vi "Find Average Center.vi"(5 "Position":i32, 7 "Tray Number":i32, 9 "XYZTheta":dbl[](array[numeric]), 11 "Gantry In":refnum<k24>) -> (1 "XYZTheta":dbl[](array[numeric]) format="%.6g", 3 "Gantry Out":refnum<k24>)   [LabVIEW 2020, in "Component Tray.lvclass"]
uses:
  Component Tray.lvclass
  Controller/Camera/Edmund Optics/Edmund Optics.lvclass
  Controller/Camera/Camera.lvclass
  Controller/Motion/A3200/A3200.lvclass
  Controller/Motion/Motion.lvclass
  Find Component.ctl
  Controller/Camera/Machine Vision.ctl
  C:/Program Files (x86)/Aerotech/A3200/LabVIEW/2010/Bin/Aerotech.A3200.dll
  Program Files (x86)/Aerotech/A3200/LabVIEW/2010/Bin/Aerotech.A3200.dll
  Controller/Camera/Camera settings.ctl
  Controller/Camera/Image processing.ctl
  Controller/Camera/Material.ctl
panel:
  out "Program Stopped":bool
  out "XY Graph":cluster{"X":dbl, "Y":dbl}[](graph)
  out "Sensor ID Location":dbl[](array[numeric])
  in  "Go to Sensor ID":bool
  out "CH1 Location":dbl[](array[numeric])
  in  "Verify CH1":bool
  out "CH1 correct?":bool
  in  "Go to CH1":bool
  in  "Focus step size":dbl format="%#_13g"
  in  "number of focus steps":i32
  out "Average Strength":dbl
  in  "Focus":bool
  in  "Material":T1
  out "All fiducials recorded":bool
  in  "Override presets":bool
  in  "Camera settings":T2={"Gamma"=1.6, "Gain"=0, "Sharpness"=0, "Contrast"=0.0, "Exposure"=0.0078125} {"Exposure" min=0.000244140625 max=0.5 scale=0.0002..0.5; "Contrast" min=0.0 max=1.0 scale=0.001..1.0; "Sharpness" min=0 max=2 step=1 scale=0.0..2.0; "Gain" min=0 max=100 step=1 scale=0.1..100.0; "Gamma" min=0.01 max=10.0 scale=0.01..10.0}
  in  "Image processing":T3={"Brightness"=128.0, "Contrast"=45.0, "Gamma"=1.0471123} {"Brightness" scale=0.0..400.0; "Contrast" scale=0.0..90.0; "Gamma" scale=0.005..5.0}
  in  "Machine Vision":T4
  out "Gantry":dbl[](array[numeric]) format="%.6g"
  out "Sum":dbl[](array[numeric]) format="%.6g"
  out "CH197 XY":dbl[](array[numeric]) format="%.6g"
  out "CH7 XY":dbl[](array[numeric]) format="%.6g"
  out "CH191 XY":dbl[](array[numeric]) format="%.6g"
  out "CH2 XY":dbl[](array[numeric]) format="%.6g"
  in  "Record CH7":bool
  in  "Record CH197":bool
  in  "Record CH191":bool
  in  "Record CH2":bool
  in  "Go to CH197":bool
  in  "Go to CH7":bool
  in  "Go to CH191":bool
  in  "Go to CH2":bool
  in  "Joystick":bool
  out "Camera":dbl[](array[numeric]) format="%.6g"
  in  "Go to Center":bool
  in  "Component":T5
  in  "Stop Program":bool
  out "Image":T6(plugin-control)
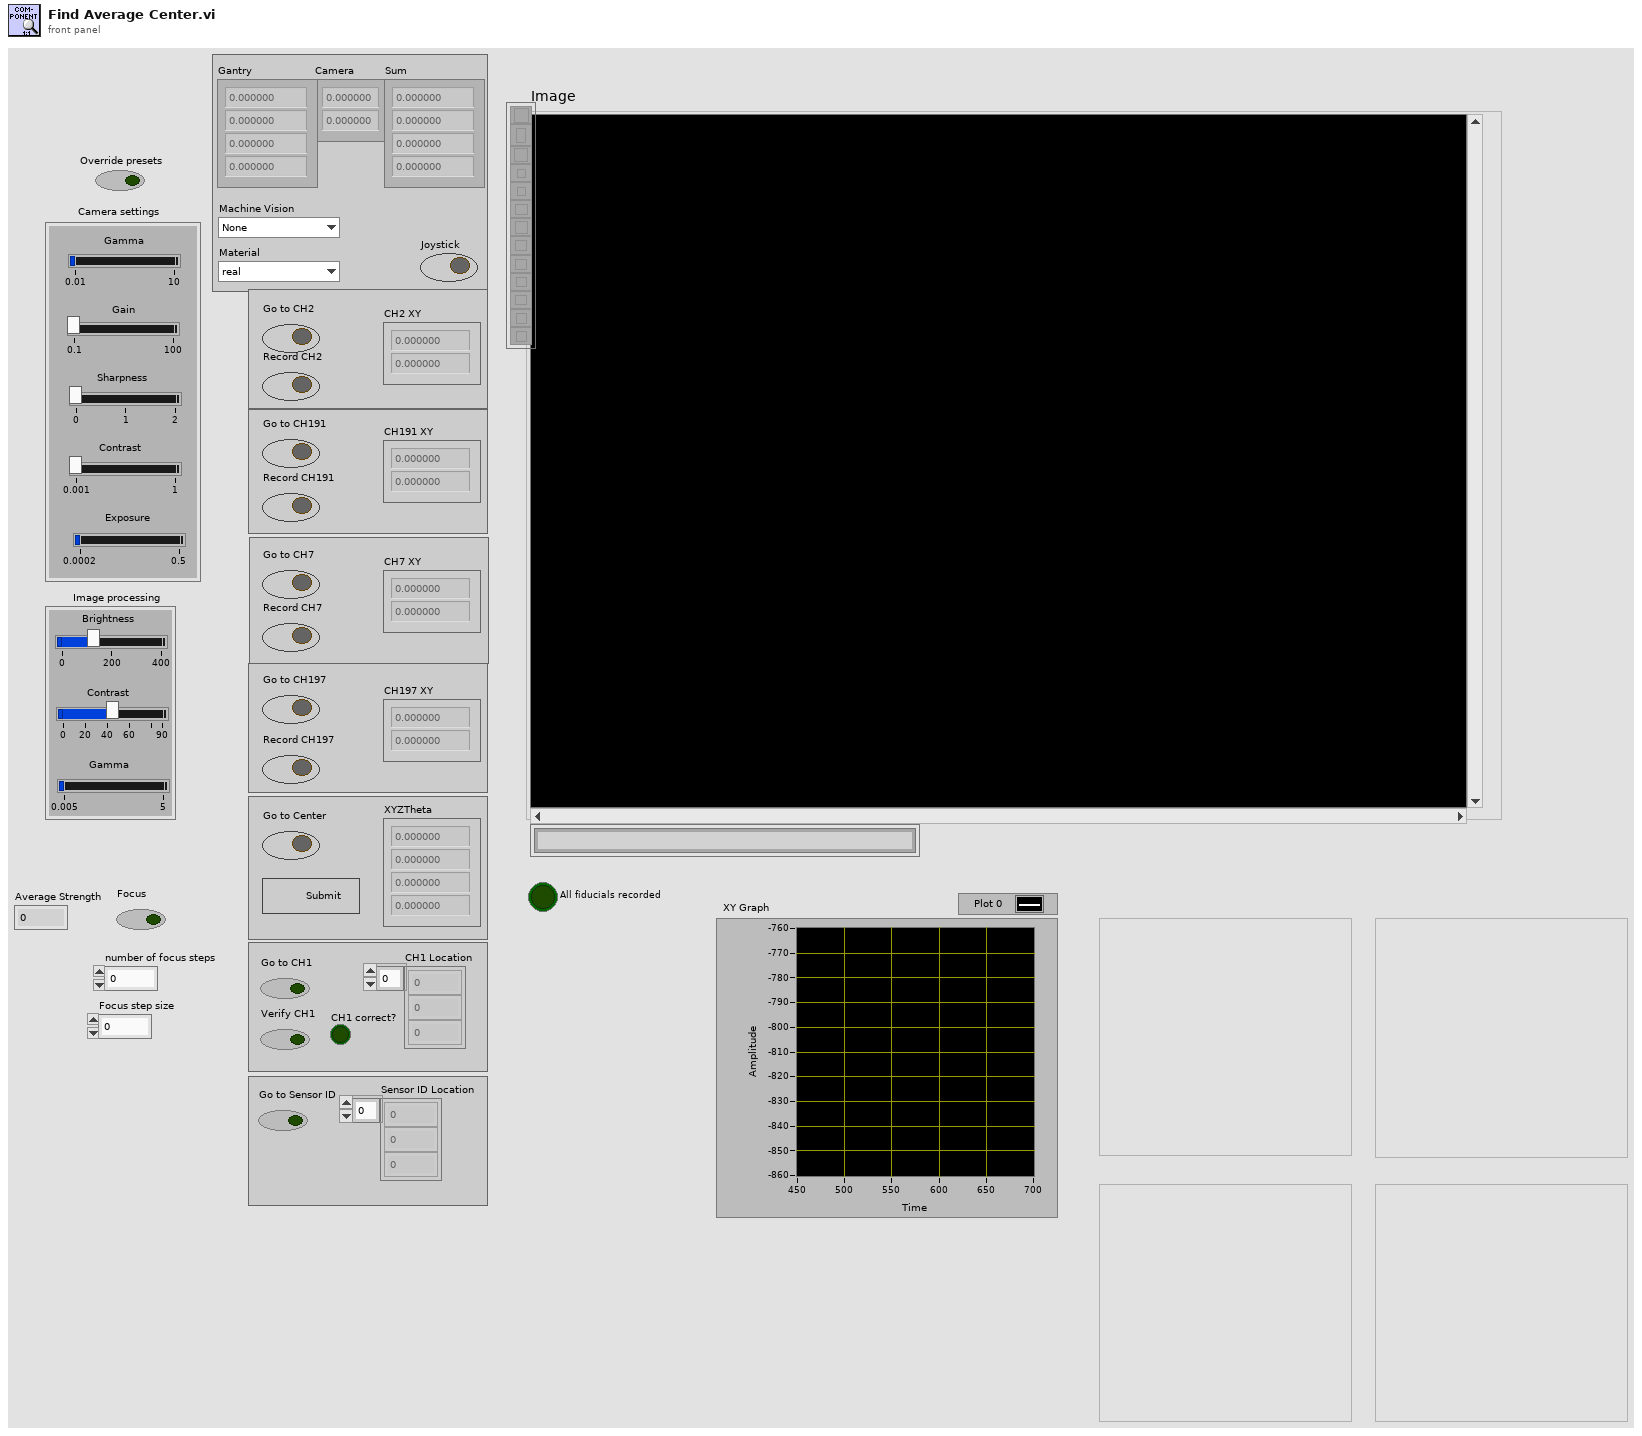
[diagram p1: front panel]
types:
  T1 = typedef "Camera.lvclass/Material.ctl" = enum16{"real", "dummy", "PETG"}
  T2 = typedef "Camera.lvclass/Camera settings.ctl" = cluster{"Gamma":dbl, "Gain":i64, "Sharpness":i64, "Contrast":dbl, "Exposure":dbl}
  T3 = typedef "Camera.lvclass/Image processing.ctl" = cluster{"Brightness":sgl, "Contrast":sgl, "Gamma":sgl}
  T4 = typedef "Camera.lvclass/Machine Vision.ctl" = enum16{"None", "Tray Fiducials", "HPK Silicon", "100um dot", "Hexaboard", "Corner (TL, BR)", "Corner (BL, TR)", "BP gold pad 1", "BP gold pad 2", "BP gold pad 3", "dummy sensor CH2", "dummy sensor CH7", "dummy sensor CH191", "dummy sensor CH197", "sensor box", "sensor circle", "PCB PETG CH2", "PCB PETG CH7", "PCB PETG CH191", "PCB PETG CH197"}
  T5 = typedef "Component Tray.lvclass/Find Component.ctl" = cluster{"New Fiducials":dbl[], "Past Fiducials":dbl[], "XYZTheta":dbl[], "Fiducials Path":path, "Position":i32, "CH1 Location":dbl[], "Sensor ID Location":dbl[]}
  T6 = typedef "IMAQ Image.ctl" = refnum<image>
  T7 = typedef "File Paths.ctl" = cluster{"Glue Pattern Folder":path, "Carrier Tray Folder":path, "Pick Up Tool Fixture Folder":path, "Components Folder":path, "Bellows Tool Offset.txt":path, "Pick Up Tool Offset.txt":path, "Dispense Tip Offset.txt":path, "Log Files":path, "Gantry Assembly Map.txt":path, "Syringe and offset map.txt":path}
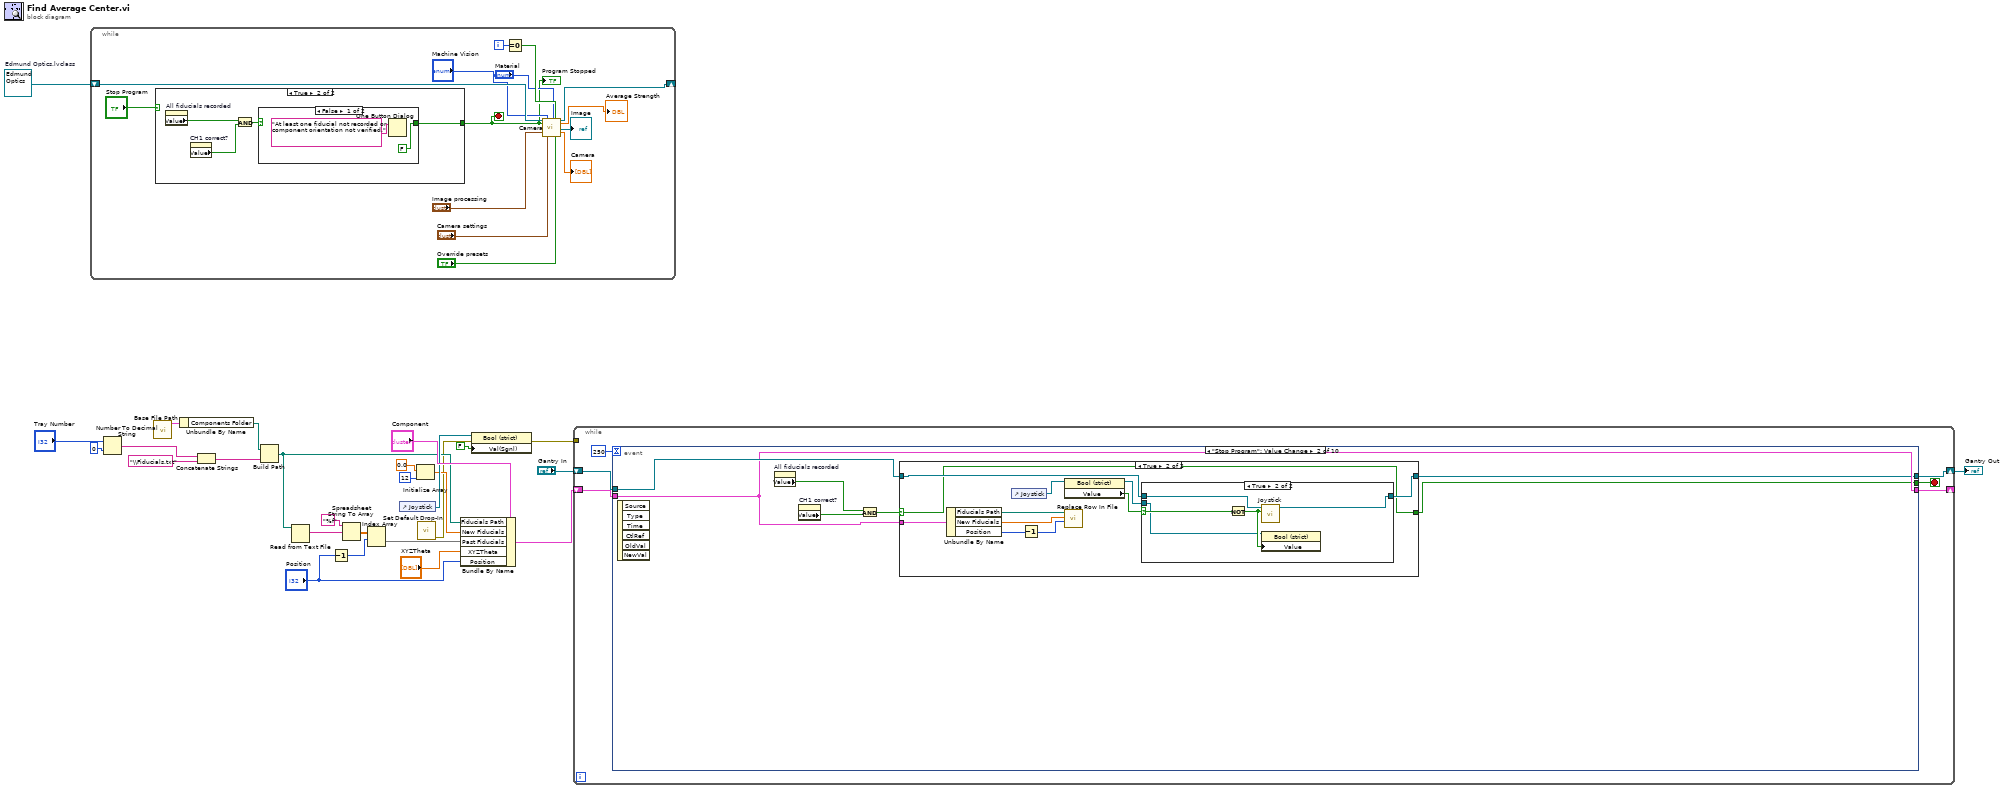
[diagram p0: block diagram]
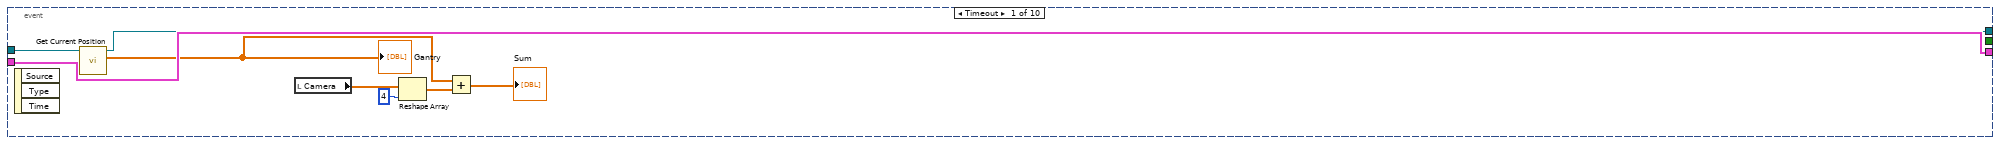
[diagram p2: hidden frame]
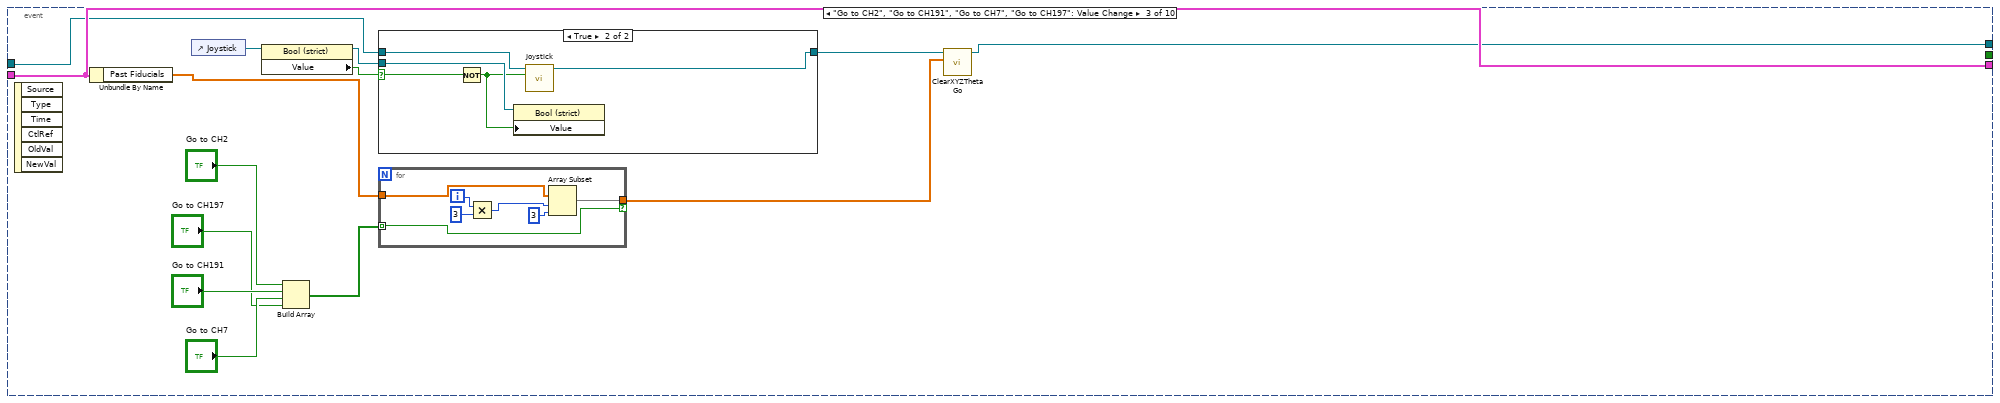
[diagram p5: hidden frame]
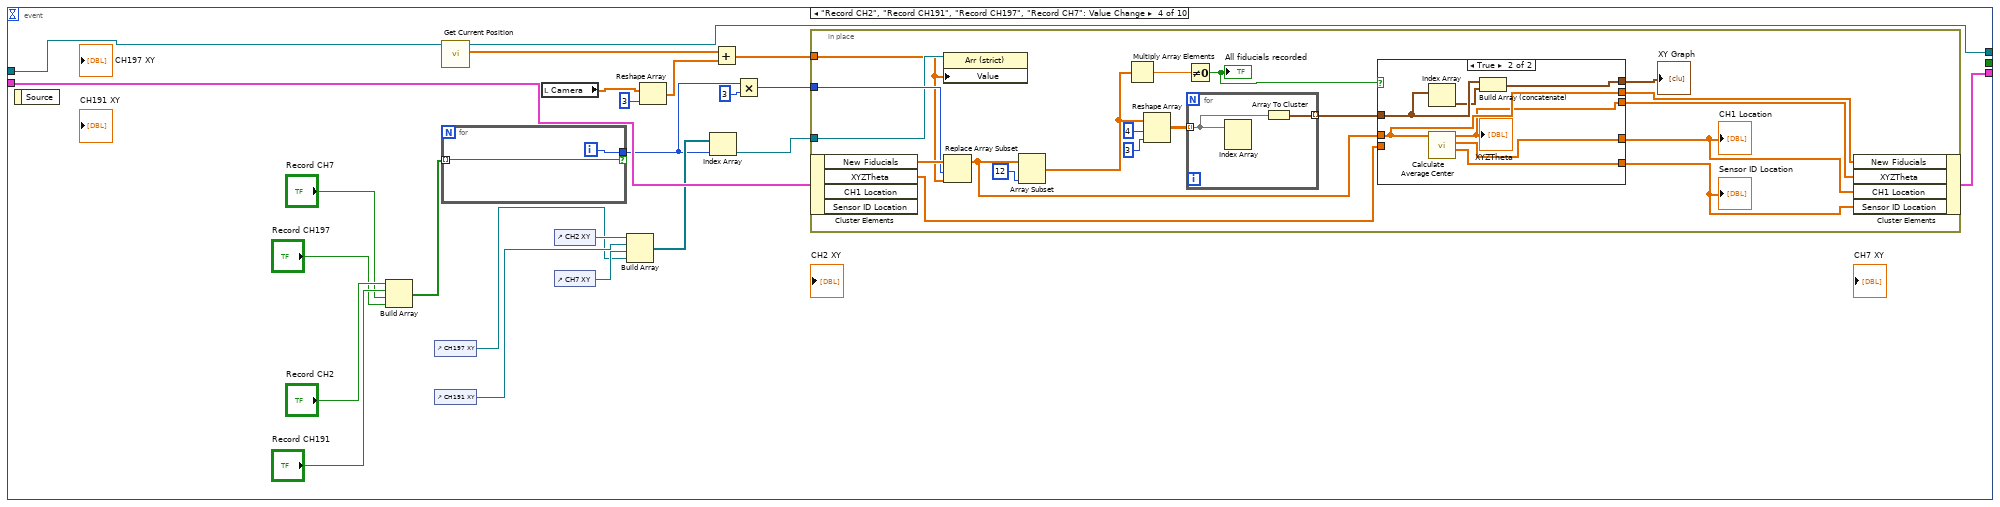
[diagram p7: hidden frame]
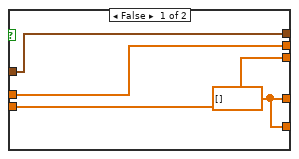
[diagram p8: hidden frame]
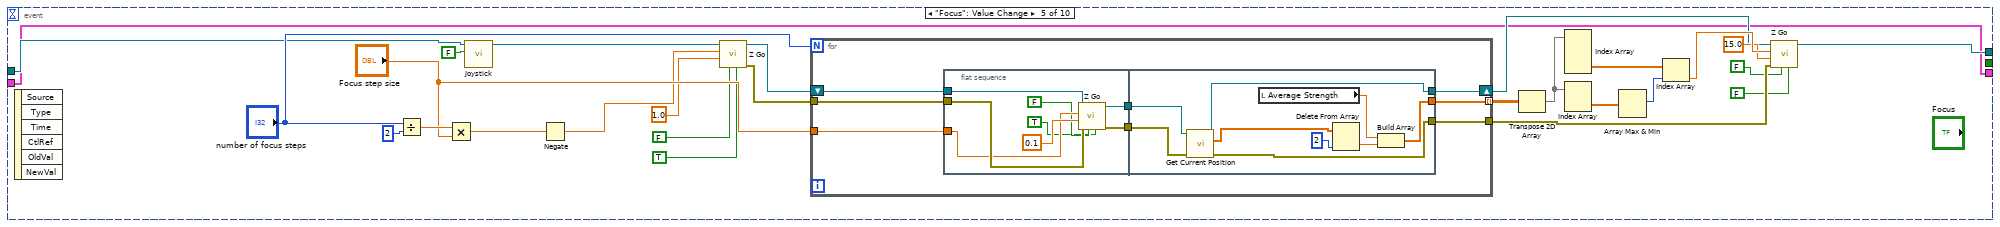
[diagram p9: hidden frame]
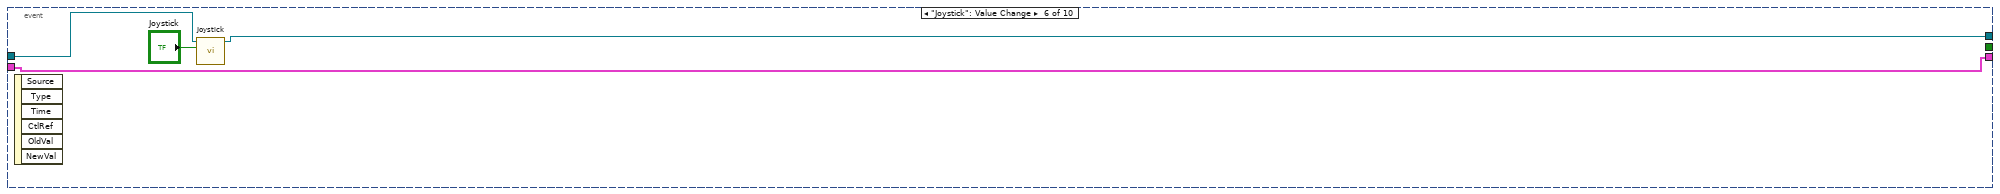
[diagram p10: hidden frame]
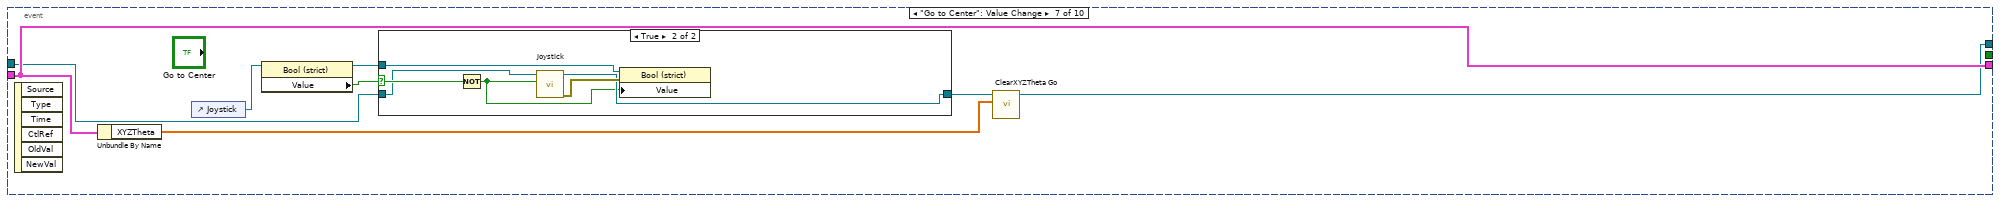
[diagram p11: hidden frame]
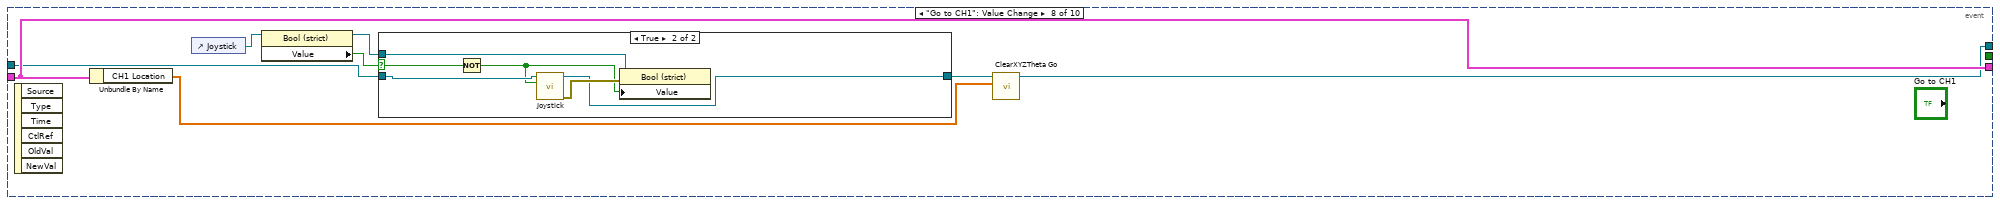
[diagram p13: hidden frame]
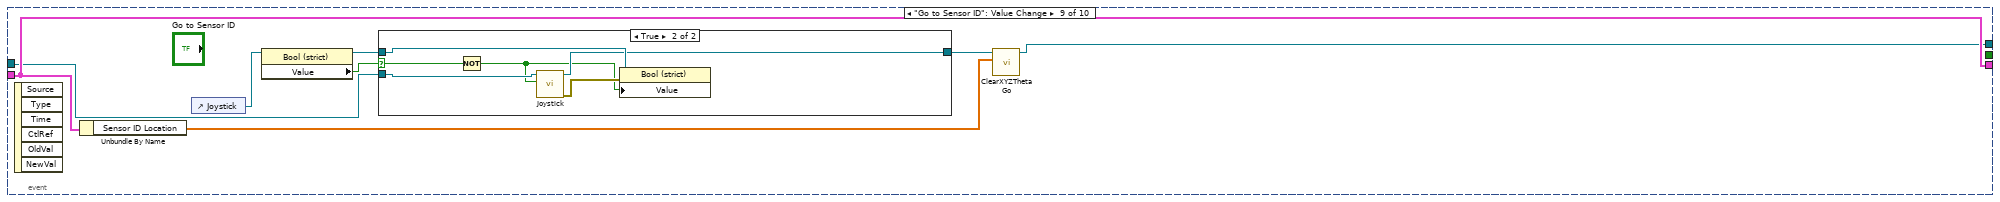
[diagram p15: hidden frame]
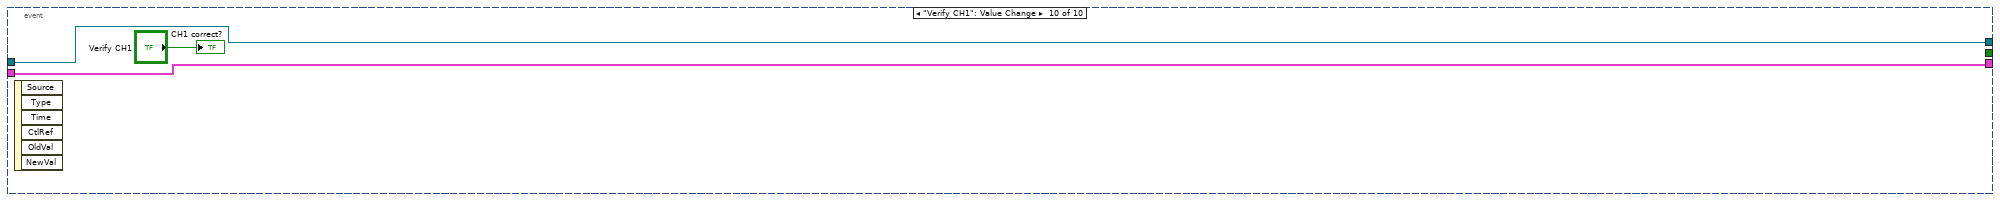
[diagram p17: hidden frame]
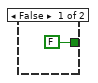
[diagram p18: hidden frame]
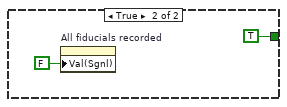
[diagram p19: hidden frame]
diagram:
  w22 = refnum<class "Edmund Optics.lvclass"> refnum  # Edmund Optics.lvclass
  n1 = while {
    shift-right: [w37] -> _
    shift-left: w22 -> [w41]
    i -> [w33]
    stop <- w28 stop-if-true
    n2 = case shown="True" "Stop Program" {
      tunnel: [FALSE w43] -> w28
      frame False {
      }
      frame True {
        n3 = property on="All fiducials recorded" class="Bool (strict)"() -> ("Value"=w46:bool)  [unwired: 2 in, 2 out]
        n4 = property on="CH1 correct?" class="Bool (strict)"() -> ("Value"=w44:bool)  [unwired: 2 in, 2 out]
        n5 = And(x=w46, y=w44) -> (x .and. y?=w45:bool)
        n6 = case shown="False" w45 {
          tunnel: [FALSE TRUE] -> w43
          frame False {
            n7 = One Button Dialog(message="At least one fiducial not recorded or component orientation not verified.") -> ()  [unwired: 1 in, 1 out]
          }
          frame True {
            n8 = property on="All fiducials recorded" class="Bool (strict)"("Val(Sgnl)"=FALSE) -> ()  [unwired: 2 in, 2 out]
          }
        }
      }
    }
    "Program Stopped" <- w28
    n9 = Equal To 0?(x=w33) -> (x = 0?=w32:bool)
    n10 = call "Camera.vi"("Camera in"=w41, "Stop"=w28, "BCG Image Processing"="Image processing", "Machine Vision"="Machine Vision", "Camera settings"="Camera settings", "Material"="Material", "Loop 0"=w32, "Override presets"="Override presets") -> ("Camera out"=w37:refnum<class "Edmund Optics.lvclass">, "Average Strength"=→"Average Strength":dbl, "Image"=→"Image":T6, "Camera"=→"Camera":dbl[])  [unwired: 6 in, 2 out]
  }
  n11 = Number To Decimal String(number="Tray Number", width (-)=i16 0) -> (decimal integer string=w16:string)
  n12 = call "Base File Path.vi"() -> ("Paths Out"=w13:T7)  [unwired: 11 in]
  n13 = Unbundle By Name(w13) -> ("Components Folder"=w15:path)
  n14 = Concatenate Strings(w16, "\\Fiducials.txt" ("string")) -> (w18:string)
  n15 = Build Path(base path=w15, name or relative path=w18) -> (appended path=w7:path)
  n16 = Read from Text File(file (use dialog)=w7) -> (text=w19:string)  [unwired: 3 in, 3 out]
  n17 = Decrement(x="Position") -> (x-1=w4:i32)
  n18 = Spreadsheet String To Array(format string="%f", spreadsheet string=w19) -> (array=w21:dbl[][])  [unwired: 2 in]
  n19 = Index Array(array=w21, index (row)=w4) -> (element=w11:dbl[])  [unwired: 1 in]
  n20 = control-ref of="Joystick"() -> (w25:refnum<vi>)
  n21 = Initialize Array(0.0 ("element"), 12 ("dimension size")) -> (w10:dbl[])
  n22 = call "Set Default Drop-In.vi"() -> ("error out"=w3:errorcluster)  [unwired: 11 in]
  n23 = Bundle By Name(cluster="Component", "Fiducials Path"=w7, "New Fiducials"=w10, "Past Fiducials"=w11, "XYZTheta"="XYZTheta", "Position"="Position") -> (w26:T5)
  n24 = property class="Bool (strict)"(reference=w25, error in=w3, "Val(Sgnl)"=FALSE) -> (error out=w23:errorcluster)  [unwired: 1 out]
  n25 = while {
    shift-right: [w54] -> _
    shift-left: w26 -> [w55]
    tunnel: w23 -> [_]
    shift-right: [w51] -> w1
    shift-left: "Gantry In" -> [w52]
    stop <- w56 stop-if-true
    n26 = event shown="[1] \"Stop Program\": Value Change" {
      selector: _ -> [_ _ _ _ _ _ _ _ _ _]
      dyn-events: _ -> [_ _ _ _ _ _ _ _ _ _]
      timeout: 250 -> [_ _ _ _ _ _ _ _ _ _]
      tunnel: [_ w68 _ _ _ _ _ _ _ _] -> w56
      tunnel: w55 -> [w63 w70 w97 w140 w184 w230 w237 w252 w267 w277]
      tunnel: [w63 w70 w97 w139 w184 w230 w237 w252 w267 w277] -> w54
      tunnel: w52 -> [w59 w71 w94 w120 w186 w229 w233 w248 w263 w278]
      tunnel: [w58 w69 w91 w118 w185 w227 w231 w246 w261 w278] -> w51
      event Timeout {
        n27 = event-data() -> ()  [unwired: 1 in, 3 out]
        n28 = call "Get Current Position.vi"("Gantry In"=w59) -> ("XYZTheta Out"=w57:dbl[], "Gantry Out"=w58:refnum<k24>)  [unwired: 8 in, 1 out]
        "Gantry" <- w57
        n29 = local read "Camera"() -> (w62:dbl[])
        n30 = Reshape Array(w62, 4 ("dimension size")) -> (w60:dbl[])
        n31 = Add(x=w57, y=w60) -> (x+y=→"Sum":dbl[])
      }
      event "Stop Program": Value Change {
        n32 = event-data() -> ()  [unwired: 1 in, 6 out]
        n33 = property on="All fiducials recorded" class="Bool (strict)"() -> ("Value"=w66:bool)  [unwired: 2 in, 2 out]
        n34 = property on="CH1 correct?" class="Bool (strict)"() -> ("Value"=w67:bool)  [unwired: 2 in, 2 out]
        n35 = And(x=w66, y=w67) -> (x .and. y?=w65:bool)
        n36 = case shown="True" w65 {
          selector: w65 -> [w72 w81]
          tunnel: w71 -> [w73 w83]
          tunnel: w70 -> [_ w84]
          tunnel: [w73 w82] -> w69
          tunnel: [w72 w81] -> w68
          frame False {
          }
          frame True {
            n37 = Unbundle By Name(w84) -> ("Fiducials Path"=w78:path, "New Fiducials"=w77:dbl[], "Position"=w79:i32)
            n38 = control-ref of="Joystick"() -> (w75:refnum<vi>)
            n39 = Decrement(x=w79) -> (x-1=w80:i32)
            n40 = property class="Bool (strict)"(reference=w75) -> (reference out=w74:refnum<vi>, "Value"=w76:bool)  [unwired: 1 in, 1 out]
            n41 = call "Replace Row In File.vi"("Index"=w80, "Insert Array"=w77, "Path"=w78) -> ()  [unwired: 8 in, 1 out]
            n42 = case shown="True" w76 {
              selector: w76 -> [_ w90]
              tunnel: w83 -> [w85 w89]
              tunnel: [w85 w88] -> w82
              tunnel: w74 -> [_ w86]
              frame False {
              }
              frame True {
                n43 = Not(x=w90) -> (.not. x?=w87:bool)
                n44 = call "Joystick.vi"("Joystick"=w87, "Gantry In"=w89) -> ("Gantry Out"=w88:refnum<k24>)  [unwired: 8 in, 1 out]
                n45 = property class="Bool (strict)"(reference=w86, "Value"=w87) -> ()  [unwired: 1 in, 2 out]
              }
            }
          }
        }
      }
      event "Go to CH2", "Go to CH191", "Go to CH7", "Go to CH197": Value Change {
        n46 = event-data() -> ()  [unwired: 1 in, 6 out]
        n47 = Unbundle By Name(w97) -> ("Past Fiducials"=w99:dbl[])
        n48 = control-ref of="Joystick"() -> (w92:refnum<vi>)
        n49 = property class="Bool (strict)"(reference=w92) -> (reference out=w95:refnum<vi>, "Value"=w96:bool)  [unwired: 1 in, 1 out]
        n50 = Build Array("Go to CH2", "Go to CH191", "Go to CH7", "Go to CH197") -> (w100:bool[])
        n51 = case shown="True" w96 {
          selector: w96 -> [_ w110]
          tunnel: w94 -> [w105 w108]
          tunnel: [w105 w106] -> w93
          tunnel: w95 -> [_ w109]
          frame False {
          }
          frame True {
            n52 = Not(x=w110) -> (.not. x?=w107:bool)
            n53 = property class="Bool (strict)"(reference=w109, "Value"=w107) -> ()  [unwired: 1 in, 2 out]
            n54 = call "Joystick.vi"("Joystick"=w107, "Gantry In"=w108) -> ("Gantry Out"=w106:refnum<k24>)  [unwired: 8 in, 1 out]
          }
        }
        n55 = for {
          tunnel: w100 -> [w117] mode=indexing
          tunnel: w99 -> [w116]
          tunnel: [w111] -> w98 if=w117
          i -> [w114]
          n56 = Multiply(x=w114, y=3) -> (x*y=w112:i32)
          n57 = Array Subset(array=w116, index=w112, length=3) -> (w111:dbl[])
        }
        n58 = call "ClearXYZTheta Go.vi"("XYZTheta In"=w98, "Gantry In"=w93) -> ("Gantry Out"=w91:refnum<k24>)  [unwired: 7 in, 2 out]
      }
      event "Record CH2", "Record CH191", "Record CH197", "Record CH7": Value Change {
        n59 = event-data() -> ()  [unwired: 1 in, 1 out]
        n60 = Build Array("Record CH2", "Record CH191", "Record CH7", "Record CH197") -> (w134:bool[])
        n61 = control-ref of="CH197 XY"() -> (w130:refnum<vi>)
        n62 = control-ref of="CH191 XY"() -> (w132:refnum<vi>)
        n63 = call "Get Current Position.vi"("Gantry In"=w120) -> ("XYZTheta Out"=w119:dbl[], "Gantry Out"=w118:refnum<k24>)  [unwired: 8 in, 1 out]
        n64 = for {
          tunnel: w134 -> [w141] mode=indexing
          tunnel: [w142] -> w126 if=w141
          i -> [w142]
        }
        n65 = local read "Camera"() -> (w123:dbl[])
        n66 = control-ref of="CH2 XY"() -> (w133:refnum<vi>)
        n67 = control-ref of="CH7 XY"() -> (w131:refnum<vi>)
        n68 = Build Array(w133, w132, w131, w130) -> (w129:refnum<vi>[])
        n69 = Reshape Array(w123, 3 ("dimension size")) -> (w122:dbl[])
        n70 = Index Array(array=w129, index=w126) -> (element=w128:refnum<vi>)
        n71 = Add(x=w119, y=w122) -> (x+y=w121:dbl[])
        n72 = Multiply(x=w126, y=3) -> (x*y=w124:i32)
        n73 = in-place {
          in-place-border: w124 -> [w159]
          in-place-border: w128 -> [w157]
          in-place-border: w121 -> [w155]
          n74 = in-place-cluster #1(w140) -> ("New Fiducials"=w160:dbl[], "XYZTheta"=w156:dbl[])  [unwired: 2 out]
          n75 = property class="Arr (strict)"(reference=w157, "Value"=w155) -> ()  [unwired: 1 in, 2 out]
          n76 = Replace Array Subset(array=w160, new element=w155, index=w159) -> (w154:dbl[])
          n77 = Array Subset(array=w154, length=12) -> (w149:dbl[])  [unwired: 1 in]
          n78 = Multiply Array Elements(1:w149) -> (0:w152:dbl)
          n79 = Reshape Array(w149, 4 ("dimension size"), 3 ("dimension size")) -> (w146:dbl[][])
          n80 = Not Equal To 0?(x=w152) -> (x != 0?=w143:bool)
          "All fiducials recorded" <- w143
          n81 = for {
            tunnel: w146 -> [w162] mode=indexing
            tunnel: [w163] -> w145 mode=indexing
            n82 = Index Array(array=w162) -> ()  [unwired: 2 in, 2 out]
            n83 = Array To Cluster(array=w162) -> (cluster=w163:cluster{"[0]":dbl, "[1]":dbl})
          }
          n84 = case shown="True" w143 {
            tunnel: [w166 w173] -> w161
            tunnel: w154 -> [w167 w174]
            tunnel: [w167 w174] -> w158
            tunnel: w156 -> [w166 _]
            tunnel: [w165 w172] -> w151
            tunnel: [w165 w171] -> w150
            tunnel: w145 -> [w164 w170]
            tunnel: [w164 w168] -> w144
            frame False {
              w165 = dbl[] [] ("CH1 location")
            }
            frame True {
              n85 = Index Array(array=w170) -> (element=w169:cluster{"[0]":dbl, "[1]":dbl})  [unwired: 1 in]
              n86 = call "Calculate Average Center.vi"("Gantry Fiducials"=w174) -> ("Sensor ID Location"=w171:dbl[], "CH1 Location"=w172:dbl[], "XYZTheta"=w173:dbl[])  [unwired: 8 in]
              "XYZTheta" <- w173
              n87 = Build Array (concatenate)(w170, w169) -> (w168:cluster{"[0]":dbl, "[1]":dbl}[])
            }
          }
          "CH1 Location" <- w151
          "Sensor ID Location" <- w150
          "XY Graph" <- w144
          n88 = in-place-cluster #1("New Fiducials"=w158, "XYZTheta"=w161, "CH1 Location"=w151, "Sensor ID Location"=w150) -> (w139:T5)
        }
      }
      event "Focus": Value Change {
        n89 = event-data() -> ()  [unwired: 1 in, 6 out]
        n90 = Divide(x="number of focus steps", y=2) -> (x/y=w189:dbl)
        n91 = Multiply(x=w189, y="Focus step size") -> (x*y=w187:dbl)
        n92 = call "Joystick.vi"("Joystick"=FALSE, "Gantry In"=w186) -> ("Gantry Out"=w180:refnum<k24>)  [unwired: 8 in, 1 out]
        n93 = Negate(x=w187) -> (-x=w181:dbl)
        n94 = call "Z Go.vi"("Increment"=TRUE, "Return Immediately"=FALSE ("Increment"), "Speed In"=1.0 ("Speed"), "Position In"=w181, "Gantry In"=w180) -> ("error out"=w178:errorcluster, "Gantry Out"=w179:refnum<k24>)  [unwired: 3 in, 2 out]
        n95 = for {
          N: "number of focus steps" -> [_]
          tunnel: [w206] -> w200 mode=indexing
          tunnel: w178 -> [w205]
          tunnel: [w203] -> w193
          shift-right: [w207] -> w194
          shift-left: w179 -> [w209]
          tunnel: "Focus step size" -> [w202]
          n96 = flat-sequence {
            tunnel: w209 -> [w217]
            tunnel: [w216] -> w208
            tunnel: w205 -> [w215]
            tunnel: [w214] -> w204
            tunnel: w202 -> [w212]
            tunnel: w208 -> [w226]
            tunnel: [w225] -> w207
            tunnel: [w224] -> w206
            tunnel: w204 -> [w220]
            tunnel: [w219] -> w203
            frame #0 {
              n97 = call "Z Go.vi"("Increment"=TRUE, "Return Immediately"=FALSE ("Increment"), "error in (no error)"=w215, "Speed In"=0.1 ("Speed"), "Position In"=w212, "Gantry In"=w217) -> ("error out"=w214:errorcluster, "Gantry Out"=w216:refnum<k24>)  [unwired: 2 in, 2 out]
            }
            frame #1 {
              n98 = call "Get Current Position.vi"("error in (no error)"=w220, "Gantry In"=w226) -> ("error out"=w219:errorcluster, "XYZTheta Out"=w223:dbl[], "Gantry Out"=w225:refnum<k24>)  [unwired: 7 in]
              n99 = local read "Average Strength"() -> (w218:dbl)
              n100 = Delete From Array(array=w223, index=2) -> (deleted portion=w221:dbl)  [unwired: 1 in, 1 out]
              n101 = Build Array(w218, w221) -> (w224:dbl[])
            }
          }
        }
        n102 = Transpose 2D Array(2D array=w200) -> (transposed array=w199:dbl[][])
        n103 = Index Array(array=w199) -> (element #2=w198:dbl[])  [unwired: 4 in, 1 out]
        n104 = Index Array(array=w199) -> (element=w201:dbl[])  [unwired: 2 in]
        n105 = Array Max & Min(array=w201) -> (max index (indices)=w197:i32)  [unwired: 3 out]
        n106 = Index Array(array=w198, index=w197) -> (element=w196:dbl)
        n107 = call "Z Go.vi"("Increment"=FALSE, "Return Immediately"=FALSE ("Increment"), "error in (no error)"=w193, "Speed In"=15.0 ("Speed"), "Position In"=w196, "Gantry In"=w194) -> ("Gantry Out"=w185:refnum<k24>)  [unwired: 2 in, 3 out]
      }
      event "Joystick": Value Change {
        n108 = event-data() -> ()  [unwired: 1 in, 6 out]
        n109 = call "Joystick.vi"("Joystick"="Joystick", "Gantry In"=w229) -> ("Gantry Out"=w227:refnum<k24>)  [unwired: 8 in, 1 out]
      }
      event "Go to Center": Value Change {
        n110 = event-data() -> ()  [unwired: 1 in, 6 out]
        n111 = Unbundle By Name(w237) -> ("XYZTheta"=w238:dbl[])
        n112 = control-ref of="Joystick"() -> (w234:refnum<vi>)
        n113 = property class="Bool (strict)"(reference=w234) -> (reference out=w235:refnum<vi>, "Value"=w236:bool)  [unwired: 1 in, 1 out]
        n114 = case shown="True" w236 {
          selector: w236 -> [_ w245]
          tunnel: w233 -> [w239 w242]
          tunnel: [w239 w241] -> w232
          tunnel: w235 -> [_ w244]
          frame False {
          }
          frame True {
            n115 = Not(x=w245) -> (.not. x?=w240:bool)
            n116 = call "Joystick.vi"("Joystick"=w240, "Gantry In"=w242) -> ("error out"=w243:errorcluster, "Gantry Out"=w241:refnum<k24>)  [unwired: 8 in]
            n117 = property class="Bool (strict)"(reference=w244, error in=w243, "Value"=w240) -> ()  [unwired: 2 out]
          }
        }
        n118 = call "ClearXYZTheta Go.vi"("XYZTheta In"=w238, "Gantry In"=w232) -> ("Gantry Out"=w231:refnum<k24>)  [unwired: 7 in, 2 out]
      }
      event "Go to CH1": Value Change {
        n119 = event-data() -> ()  [unwired: 1 in, 6 out]
        n120 = Unbundle By Name(w252) -> ("CH1 Location"=w253:dbl[])
        n121 = control-ref of="Joystick"() -> (w249:refnum<vi>)
        n122 = property class="Bool (strict)"(reference=w249) -> (reference out=w250:refnum<vi>, "Value"=w251:bool)  [unwired: 1 in, 1 out]
        n123 = case shown="True" w251 {
          selector: w251 -> [_ w260]
          tunnel: w248 -> [w254 w257]
          tunnel: [w254 w256] -> w247
          tunnel: w250 -> [_ w259]
          frame False {
          }
          frame True {
            n124 = Not(x=w260) -> (.not. x?=w255:bool)
            n125 = call "Joystick.vi"("Joystick"=w255, "Gantry In"=w257) -> ("error out"=w258:errorcluster, "Gantry Out"=w256:refnum<k24>)  [unwired: 8 in]
            n126 = property class="Bool (strict)"(reference=w259, error in=w258, "Value"=w255) -> ()  [unwired: 2 out]
          }
        }
        n127 = call "ClearXYZTheta Go.vi"("XYZTheta In"=w253, "Gantry In"=w247) -> ("Gantry Out"=w246:refnum<k24>)  [unwired: 7 in, 2 out]
      }
      event "Go to Sensor ID": Value Change {
        n128 = event-data() -> ()  [unwired: 1 in, 6 out]
        n129 = Unbundle By Name(w267) -> ("Sensor ID Location"=w268:dbl[])
        n130 = control-ref of="Joystick"() -> (w264:refnum<vi>)
        n131 = property class="Bool (strict)"(reference=w264) -> (reference out=w265:refnum<vi>, "Value"=w266:bool)  [unwired: 1 in, 1 out]
        n132 = case shown="True" w266 {
          selector: w266 -> [_ w275]
          tunnel: w263 -> [w269 w272]
          tunnel: [w269 w271] -> w262
          tunnel: w265 -> [_ w274]
          frame False {
          }
          frame True {
            n133 = Not(x=w275) -> (.not. x?=w270:bool)
            n134 = call "Joystick.vi"("Joystick"=w270, "Gantry In"=w272) -> ("error out"=w273:errorcluster, "Gantry Out"=w271:refnum<k24>)  [unwired: 8 in]
            n135 = property class="Bool (strict)"(reference=w274, error in=w273, "Value"=w270) -> ()  [unwired: 2 out]
          }
        }
        n136 = call "ClearXYZTheta Go.vi"("XYZTheta In"=w268, "Gantry In"=w262) -> ("Gantry Out"=w261:refnum<k24>)  [unwired: 7 in, 2 out]
      }
      event "Verify CH1": Value Change {
        n137 = event-data() -> ()  [unwired: 1 in, 6 out]
        "CH1 correct?" <- "Verify CH1"
      }
    }
  }
  "Gantry Out" <- w1
